vi "SetAllControlsVisibilityAndEnabledState.vi"(6 "error in (no error)":errorcluster, 8 "Enabled state (Enabled)":T2(ring), 9 "Visible (T)":bool=TRUE, 11 "Control State Array":T1[](array[typedef])) -> (0 "error out":errorcluster, 3 "Control State Array (out)":T1[](array[typedef]))   [LabVIEW 2017]
doc: "Modifies state variable of the control indicated by the reference. States are: Visible (T/F), Enabled (Enabled, Disabled, Disabled and greyed out)"
uses:
  Types/ControlAttributes.ctl
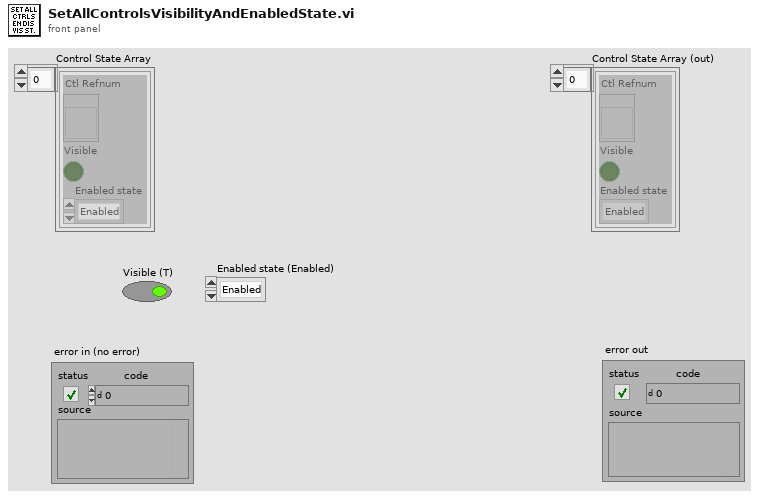
[diagram p1: front panel]
types:
  T1 = typedef "ControlAttributes.ctl" = cluster{"Ctl Refnum":refnum<vi>, "Visible":bool, "Enabled state":enum8{"Enabled", "Disabled", "Disabled and Grayed Out"}}
  T2 = enum8{"Enabled", "Disabled", "Disabled and Grayed Out"}
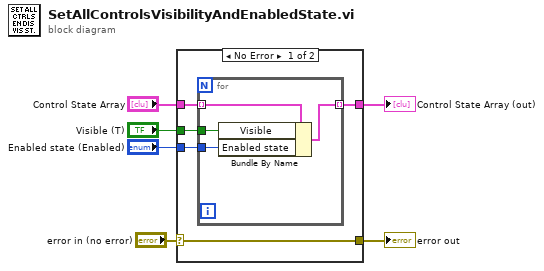
[diagram p0: block diagram]
diagram:
  n1 = case shown="No Error" "error in (no error)" {
    selector: "error in (no error)" -> [w11 w17]
    tunnel: [w11 w17] -> w5
    tunnel: "Control State Array" -> [w10 w16]
    tunnel: "Enabled state (Enabled)" -> [w9 _]
    tunnel: "Visible (T)" -> [w8 _]
    tunnel: [w7 w16] -> w1
    frame No Error {
      n2 = for {
        tunnel: w9 -> [w13]
        tunnel: w8 -> [w14]
        tunnel: w10 -> [w15] mode=indexing
        tunnel: [w12] -> w7 mode=indexing
        n3 = Bundle By Name(cluster=w15, "Visible"=w14, "Enabled state"=w13) -> (w12:T1)
      }
    }
    frame Error {
    }
  }
  "error out" <- w5
  "Control State Array (out)" <- w1
